vi "Initialization VI.vi"(8 "error in (no error)":errorcluster, 10 "Custom XML":string, 11 "Device Item Ref in":T1 format="%.0x") -> (0 "error out":errorcluster, 3 "Device Item Ref out":T1 format="%.0x")   [LabVIEW 2019, in "Diagnostics Addon System Explorer.lvlib"]
uses:
  Diagnostics Addon System Explorer.lvlib
  <vilib>/NI VeriStand/Custom Device API/Custom Device Item Ref.ctl
  <vilib>/NI VeriStand/Custom Device API/Custom Device API.lvlib
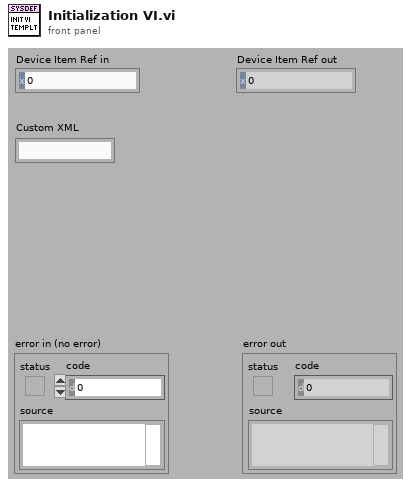
[diagram p1: front panel]
types:
  T1 = typedef "Custom Device API.lvlib/Custom Device Item Ref.ctl" = u64
  T2 = typedef "Diagnostics Addon System Explorer.lvlib/Addon.Initialize.ctl" = cluster{"Diagnostic Protocol":T3, "Previous Config":path, "Baud Rate":u32}
  T3 = typedef "Diagnostics Addon Shared.lvlib/Protocol.ctl" = enum16{"GMLAN", "KWP-2000", "UDS", "User-Defined"}
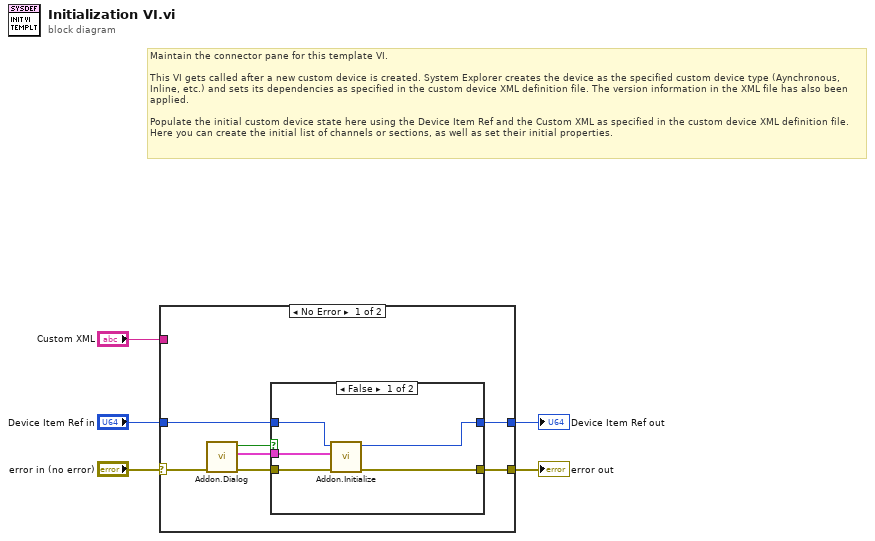
[diagram p0: block diagram]
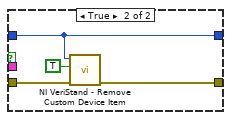
[diagram p2: hidden frame]
diagram:
  # "Maintain the connector pane for this template VI.\n\nThis VI gets called after a new custom device is created. System Explorer creates the device as the specified custom device type (Aynchronous, Inline, etc.) and sets its dependencies as specified in the custom device XML definition file. The version information in the XML file has also been applied.\n\nPopulate the initial custom device state here using the Device Item Ref and the Custom XML as specified in the custom device XML definition file. Here you can create the initial list of channels or sections, as well as set their initial properties."
  n1 = case shown="No Error" "error in (no error)" {
    selector: "error in (no error)" -> [w6 w23]
    tunnel: [w10 w23] -> w5
    tunnel: [w8 w22] -> w3
    tunnel: "Device Item Ref in" -> [w9 w22]
    tunnel: "Custom XML" -> [_ _]
    frame No Error {
      n2 = call "Addon.Dialog.vi"("error in (no error)"=w6) -> ("error out"=w11:errorcluster, "Diagnostics Basic Configuration"=w12:T2, "Cancelled?"=w7:bool)  [unwired: 8 in]
      n3 = case shown="False" w7 {
        tunnel: w12 -> [w17 _]
        tunnel: w11 -> [w13 w20]
        tunnel: [w16 w18] -> w10
        tunnel: w9 -> [w15 w19]
        tunnel: [w14 w19] -> w8
        frame False {
          n4 = call "Addon.Initialize.vi"("error in (no error)"=w13, "Diagnostics Basic Configuration"=w17, "Device Item Ref in"=w15) -> ("error out"=w16:errorcluster, "Device Item Ref out"=w14:T1)  [unwired: 7 in]
        }
        frame True {
          n5 = call <vilib>:"NI VeriStand - Remove Custom Device Item.vi"("error in (no error)"=w20, "Force Delete (F)"=TRUE, "Item Ref in"=w19) -> ("error out"=w18:errorcluster)  [unwired: 7 in, 1 out]
        }
      }
    }
    frame Error {
    }
  }
  "error out" <- w5
  "Device Item Ref out" <- w3
